vi "distance from ball to basket center.vi"(3 "d":dbl, 4 "alpha":dbl, 5 "theta":dbl) -> (0 "horizontal D2T [m]":dbl, 1 "Vertical D2T [m]":dbl, 2 "d2t":dbl)   [LabVIEW 2011]
uses:
  <vilib>/express/express arith-compare/Formula/XNode/ExpressFormulaBlockNode.xnode
panel:
  # "degrees"
  # "meters"
  # "all units are in meters and degrees"
  # "degrees"
  # "meters"
  # "t"
  # "d2t"
  # "p"
  # "w"
  # "d"
  # "fi"
  # "f"
  # "theta"
  # "h"
  # "beta"
  # "w - canon width\nh - canon height\ns - canon lowest point to camera viewing point - y\nt - distance from basket center to backboard center - y\np - distance from basket center to backboard center - x"
  # "s"
  # "alpha"
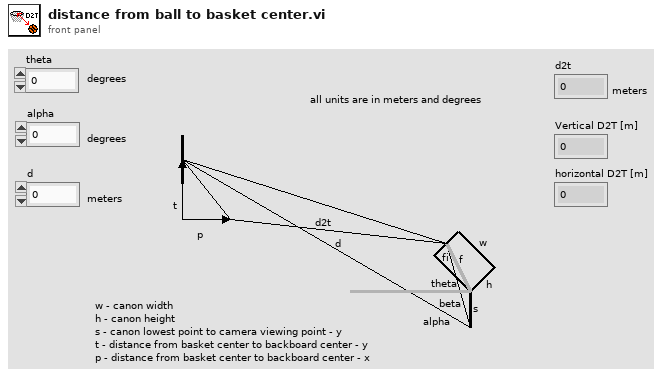
[diagram p1: front panel]
types:
  T1 = cluster{"canon height":dbl, "canon width":dbl, "distance from basket center to backboard center - x":dbl, "distance from basket center to backboard center - y":dbl, "canon lowest point to camera viewing point - y":dbl}
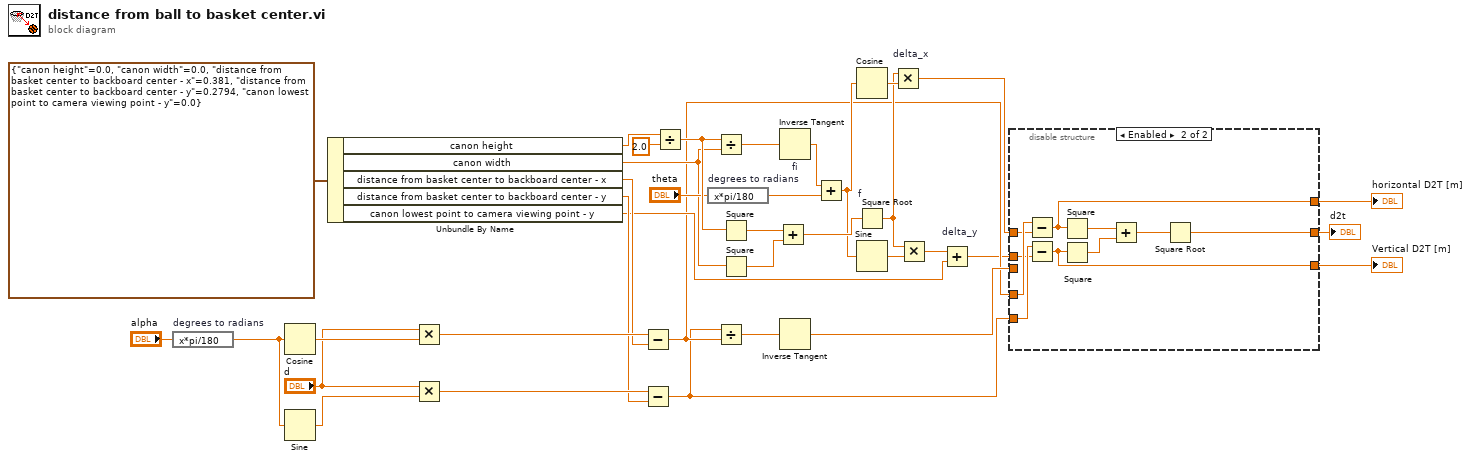
[diagram p0: block diagram]
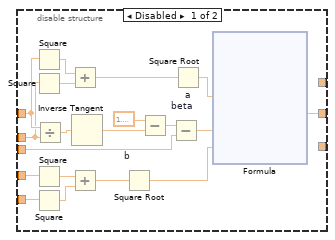
[diagram p2: hidden frame]
diagram:
  n1 = expression code="x*pi/180" "degrees to radians"("alpha") -> (w9:dbl)
  n2 = Cosine(x=w9) -> (cos(x)=w22:dbl)
  n3 = Sine(x=w9) -> (sin(x)=w20:dbl)
  n4 = Unbundle By Name(T1 {"canon height"=0.0, "canon width"=0.0, "distance from basket center to backboard center - x"=0.381, "distance from basket center to backboard center - y"=0.2794, "canon lowest point to camera viewing point - y"=0.0}) -> ("canon height"=w16:dbl, "canon width"=w15:dbl, "distance from basket center to backboard center - x"=w14:dbl, "distance from basket center to backboard center - y"=w13:dbl, "canon lowest point to camera viewing point - y"=w8:dbl)
  n5 = Multiply(x="d", y=w22) -> (x*y=w18:dbl)
  n6 = Multiply(x="d", y=w20) -> (x*y=w19:dbl)
  n7 = Subtract(x=w18, y=w14) -> (x-y=w7:dbl)
  n8 = Subtract(x=w19, y=w13) -> (x-y=w5:dbl)
  n9 = Divide(x=w16, y=2.0) -> (x/y=w32:dbl)
  n10 = expression code="x*pi/180" "degrees to radians"("theta") -> (w28:dbl)
  n11 = Divide(x=w32, y=w15) -> (x/y=w31:dbl)
  n12 = Divide(x=w5, y=w7) -> (x/y=w12:dbl)
  n13 = Square(x=w32) -> (x^2=w35:dbl)
  n14 = Square(x=w15) -> (x^2=w34:dbl)
  n15 = Add(x=w35, y=w34) -> (x+y=w33:dbl)
  n16 = Inverse Tangent "fi"(1:w31) -> (0:w30:dbl)
  n17 = Inverse Tangent ("fi")(1:w12) -> (0:w11:dbl)
  n18 = Add(x=w30, y=w28) -> (x+y=w27:dbl)
  n19 = Cosine(x=w27) -> (cos(x)=w26:dbl)
  n20 = Square Root "f"(x=w33) -> (sqrt(x)=w25:dbl)
  n21 = Sine(x=w27) -> (sin(x)=w24:dbl)
  n22 = Multiply "delta_x"(x=w25, y=w26) -> (x*y=w6:dbl)
  n23 = Multiply(x=w25, y=w24) -> (x*y=w23:dbl)
  n24 = Add "delta_y"(x=w23, y=w8) -> (x+y=w4:dbl)
  n25 = disable-structure shown="Enabled" {
    disable-tunnel: w11 -> [w48 _]
    disable-tunnel: w7 -> [w41 w73]
    disable-tunnel: w6 -> [w40 w72]
    disable-tunnel: w5 -> [w39 w71]
    disable-tunnel: w4 -> [w38 w70]
    disable-tunnel: [w37 w74] -> w3
    disable-tunnel: [_ w69] -> w2
    disable-tunnel: [_ w68] -> w1
    frame Disabled {
      n26 = Square(x=w40) -> (x^2=w47:dbl)
      n27 = Square(x=w38) -> (x^2=w46:dbl)
      n28 = Square(x=w41) -> (x^2=w52:dbl)
      n29 = Square(x=w39) -> (x^2=w51:dbl)
      n30 = Divide(x=w40, y=w38) -> (x/y=w55:dbl)
      n31 = Add(x=w47, y=w46) -> (x+y=w45:dbl)
      n32 = Add(x=w52, y=w51) -> (x+y=w50:dbl)
      n33 = Inverse Tangent ("fi")(1:w55) -> (0:w53:dbl)
      n34 = Square Root "b"(x=w50) -> (sqrt(x)=w42:dbl)
      n35 = Subtract(x=1.5707963267948966, y=w53) -> (x-y=w49:dbl)
      n36 = Subtract "beta"(x=w49, y=w48) -> (x-y=w44:dbl)
      n37 = Square Root "a"(x=w45) -> (sqrt(x)=w43:dbl)
      n38 = xnode "Formula"("a"=w43, "beta"=w44, "b"=w42) -> ("Result"=w37:dbl)  [unwired: 1 in, 1 out]
    }
    frame Enabled {
      n39 = Subtract(x=w73, y=w72) -> (x-y=w69:dbl)
      n40 = Subtract(x=w71, y=w70) -> (x-y=w68:dbl)
      n41 = Square(x=w69) -> (x^2=w75:dbl)
      n42 = Square(x=w68) -> (x^2=w76:dbl)
      n43 = Add(x=w75, y=w76) -> (x+y=w77:dbl)
      n44 = Square Root(x=w77) -> (sqrt(x)=w74:dbl)
    }
  }
  "d2t" <- w3
  "horizontal D2T [m]" <- w2
  "Vertical D2T [m]" <- w1
